vi "Set Marker Polarity.vi"(8 "error in (no error)":errorcluster {"code" format="%.0x"}, 9 "MarkerPolarity (Positive)":i32(ring) items=["Positive", "Negative"], 10 "MarkerIndex (Ss Digital Modulation Arb Marker Index One)":i32(ring) items=["Ss Digital Modulation Arb Marker Index One", "Ss Digital Modulation Arb Marker Index Two", "Ss Digital Modulation Arb Marker Index Three", "Ss Digital Modulation Arb Marker Index Four", "Ss Digital Modulation Arb Marker Index All", "Ss Digital Modulation Arb Marker Index None"], 11 "instrument handle":refnum<k15>) -> (0 "error out":errorcluster {"code" format="%.0x"}, 3 "instrument handle out":refnum<k15>)   [LabVIEW 2009, in "Keysight XSAn.lvlib"]
doc: "Set the polarity of marker.\n\nSupported Models: M8920A, M9420A, M9421A ."
uses:
  <instrlib>/Keysight XSAn/Keysight XSAn.lvlib
  AgXSAn.dll
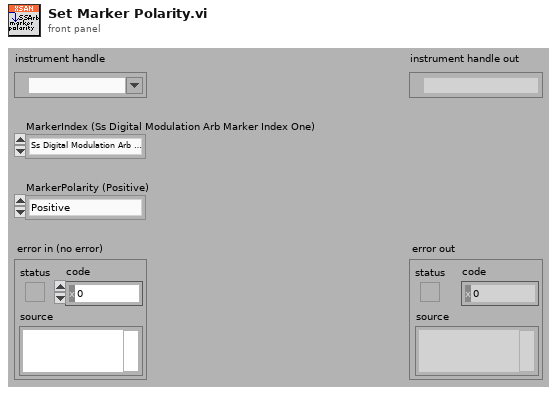
[diagram p1: front panel]
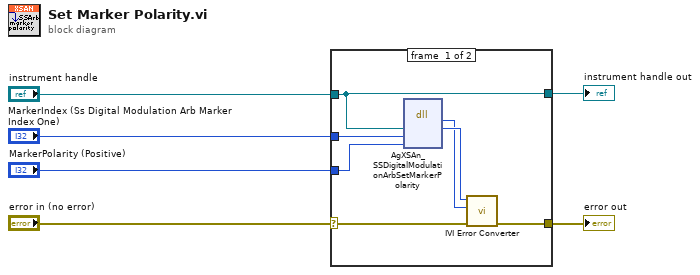
[diagram p0: block diagram]
diagram:
  n1 = case shown="No Error" "error in (no error)" {
    selector: "error in (no error)" -> [w11 w15]
    tunnel: [w10 w15] -> w6
    tunnel: "instrument handle" -> [w7 w14]
    tunnel: "MarkerIndex (Ss Digital Modulation Arb Marker Index One)" -> [w9 _]
    tunnel: "MarkerPolarity (Positive)" -> [w8 _]
    tunnel: [w7 w14] -> w1
    frame #0 {
      n2 = dll-call lib="AgXSAn**.dll" fn="AgXSAn_SSDigitalModulationArbSetMarkerPolarity"("Vi"=w7, "MarkerIndex"=w9, "MarkerPolarity"=w8) -> ("return type"=w12:i32, "Vi"=w13:u32)  [unwired: 5 in, 2 out]
      n3 = call <instrlib>:"IVI Error Converter.vi"("error in (no error)"=w11, "IVI error code (0)"=w12, "instrument handle"=w13) -> ("error out"=w10:errorcluster)  [unwired: 7 in, 1 out]
    }
    frame #1 {
    }
  }
  "error out" <- w6
  "instrument handle out" <- w1
